vi "Beam_Check_Positions.vi"(1 "Values":dbl[][](array[numeric]), 3 "Mode":T2(ring)) -> (0 "Values Out":dbl[][](array[numeric]) format="%.2f")   [LabVIEW 2013]
uses:
  Controls/Beam_Type.ctl
  Globals/Constants_global.vi
  Globals/Trav_pos_global.vi
panel:
  in  "Beam Type":T1 items=["Green Unshifted", "Green Shifted", "Blue Unshifted", "Blue Shifted"]
  # "X                        Y                        Z"
  # "X                    Y                 Z"
  # "Green Unshifted\nGreen Shifted\nBlue Unshifted\nBlue Shifted"
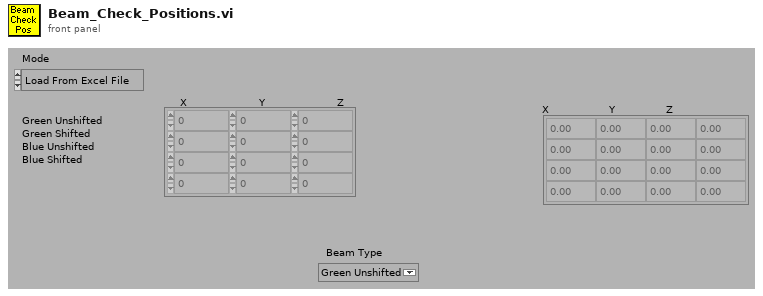
[diagram p1: front panel]
types:
  T1 = typedef "Beam_Type.ctl" = u16
  T2 = enum16{"Load From Excel File", "Save to Excel File"}
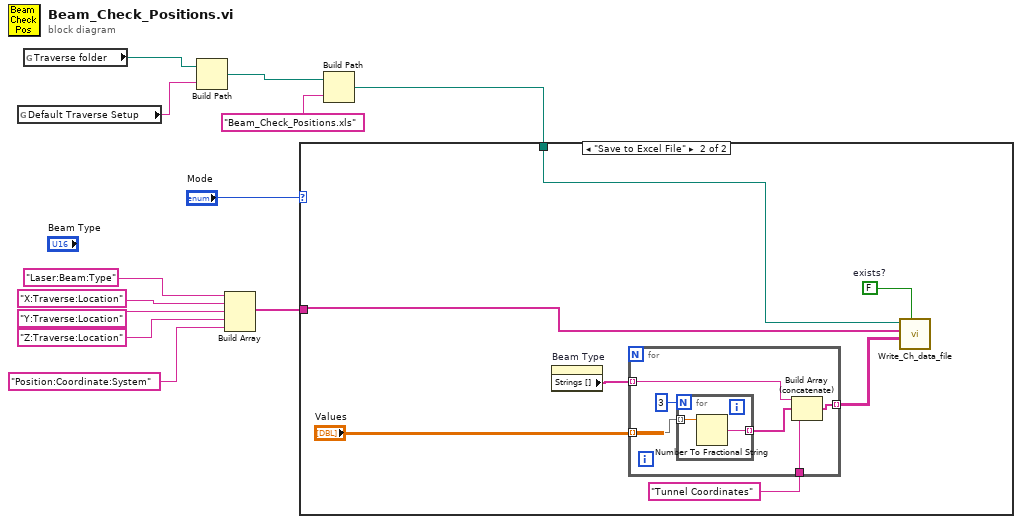
[diagram p0: block diagram]
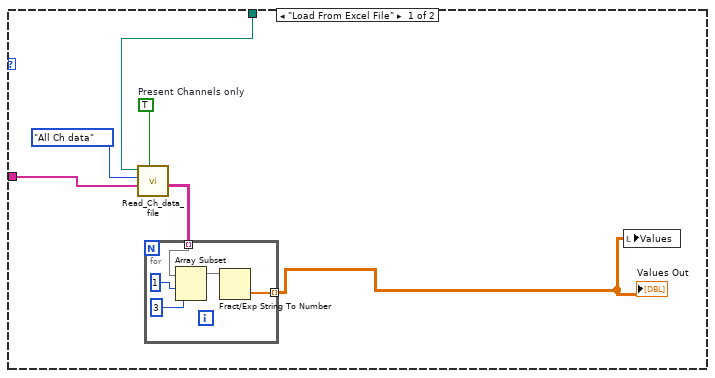
[diagram p2: hidden frame]
diagram:
  n1 = global read "Trav_pos_global.vi" "Default Traverse Setup"() -> (w2:string)
  n2 = global read "Constants_global.vi" "Traverse folder"() -> (w8:path)
  n3 = Build Path(base path=w8, name or relative path=w2) -> (appended path=w4:path)
  n4 = Build Array("Laser:Beam:Type", "X:Traverse:Location", "Y:Traverse:Location", "Z:Traverse:Location", "Position:Coordinate:System") -> (w7:string[])
  n5 = Build Path(base path=w4, name or relative path="Beam_Check_Positions.xls" ("Substring")) -> (appended path=w3:path)
  n6 = case shown="\"Save to Excel File\"" "Mode" {
    tunnel: w7 -> [w16 w28]
    tunnel: w3 -> [w15 w29]
    frame "Load From Excel File" {
      w18 = TRUE  # Present Channels only
      n7 = call "Read_Ch_data_file.vi"("Present Channels only"=w18, "Present Channels"=w16, "Output"=enum16{"All Ch data", "The last few rows"}."All Ch data", "Filename"=w15) -> ("Channel Values"=w14:string[][])  [unwired: 1 in, 4 out]
      n8 = for {
        tunnel: w14 -> [w22] mode=indexing
        tunnel: [w20] -> w13 mode=indexing
        n9 = Array Subset(array=w22, index=1 ("Array Index"), length=3) -> (w21:string[])
        n10 = Fract/Exp String To Number(string=w21) -> (number=w20:dbl[])  [unwired: 4 out]
      }
      "Values Out" <- w13
      n11 = local write "Values"(w13) -> ()
    }
    frame "Save to Excel File" {
      w30 = FALSE  # exists?
      n12 = property on="Beam Type" class="Ring (strict)"() -> ("Strings []"=w27:string[])  [unwired: 2 in, 2 out]
      n13 = for {
        tunnel: "Values" -> [w36] mode=indexing
        tunnel: w27 -> [w35] mode=indexing
        tunnel: [w33] -> w26 mode=indexing
        tunnel: "Tunnel Coordinates" -> [w32]
        n14 = for {
          N: 3 -> [_]
          tunnel: w36 -> [w38] mode=indexing
          tunnel: [w37] -> w34 mode=indexing
          n15 = Number To Fractional String(number=w38) -> (F-format string=w37:string)  [unwired: 3 out]
        }
        n16 = Build Array (concatenate)(w35, w34, w32) -> (w33:string[])
      }
      n17 = call "Write_Ch_data_file.vi"("exists?"=w30, "Channel Values"=w26, "Channel names"=w28, "Filename"=w29) -> ()  [unwired: 4 in, 4 out]
    }
  }
